vi "String.Check if is a Result Folder Name.vi"(10 "SN Len":i32=10, 11 "Name":string) -> (0 "Date":string, 1 "Time":timestamp, 2 "SN":string, 3 "OK":bool, 4 "Time":string)   [LabVIEW 2024]
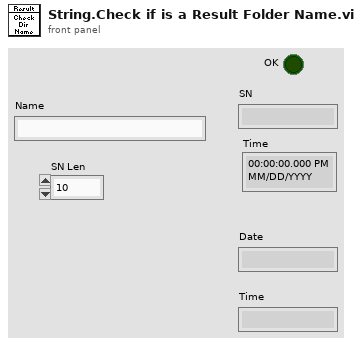
[diagram p1: front panel]
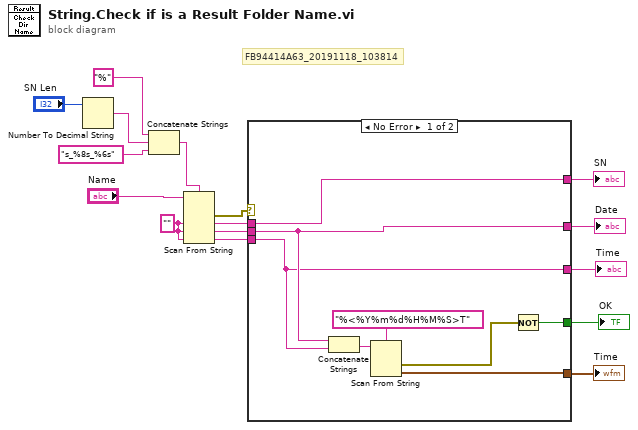
[diagram p0: block diagram]
diagram:
  w6 = "" ("default value 1")
  # "FB94414A63_20191118_103814"
  n1 = Number To Decimal String(number="SN Len") -> (decimal integer string=w1:string)  [unwired: 1 in]
  n2 = Concatenate Strings("%" ("format string"), w1, "s_%8s_%6s" ("format string")) -> (w4:string)
  n3 = Scan From String(format string=w4, input string="Name", default 1=w6, default 2=w6, default 3=w6) -> (error out=w7:errorcluster, output 1=w15:string, output 2=w14:string, output 3=w13:string)  [unwired: 2 in, 2 out]
  n4 = case shown="No Error" w7 {
    tunnel: w15 -> [w20 _]
    tunnel: w14 -> [w19 _]
    tunnel: w13 -> [w18 _]
    tunnel: [w22 _] -> w12
    tunnel: [w17 _] -> w11
    tunnel: [w20 _] -> w10
    tunnel: [w19 _] -> w9
    tunnel: [w18 _] -> w8
    frame No Error {
      n5 = Concatenate Strings(w19, w18) -> (w24:string)
      n6 = Scan From String(format string="%<%Y%m%d%H%M%S>T", input string=w24) -> (error out=w21:errorcluster, output 1=w22:timestamp)  [unwired: 3 in, 2 out]
      n7 = Not(x=w21) -> (.not. x?=w17:bool)
    }
    frame Error {
    }
  }
  "SN" <- w10
  "Time" <- w12
  "Date" <- w9
  "Time" <- w8
  "OK" <- w11
